vi "Check Lower Warning.vi"(8 "error in (no error)":errorcluster, 10 "Input Values":sgl[](array[numeric]), 11 "AILimitConfig":T1(array[cluster])) -> (0 "error out":errorcluster, 3 "LW Channel":string[](array[string]))   [LabVIEW 2018]
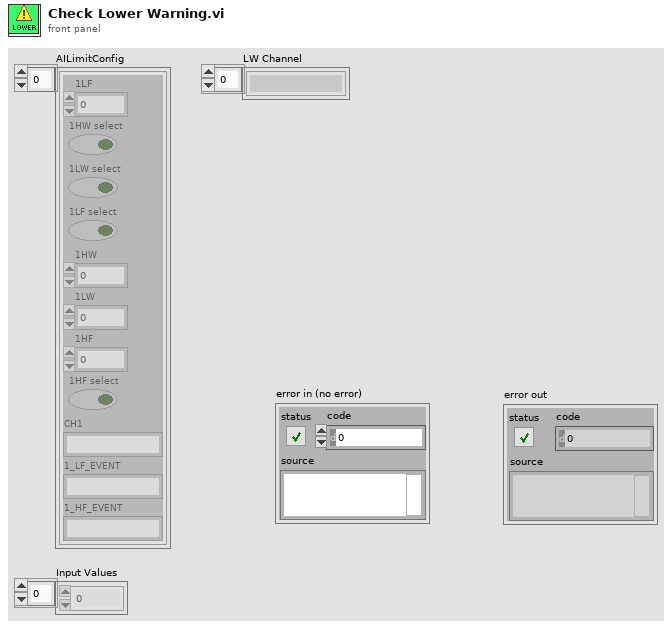
[diagram p1: front panel]
types:
  T1 = cluster{"1LF":dbl, "1HW select":bool, "1LW select":bool, "1LF select":bool, "1HW":dbl, "1LW":dbl, "1HF":dbl, "1HF select":bool, "CH1":string, "1_LF_EVENT":string, "1_HF_EVENT":string}[]
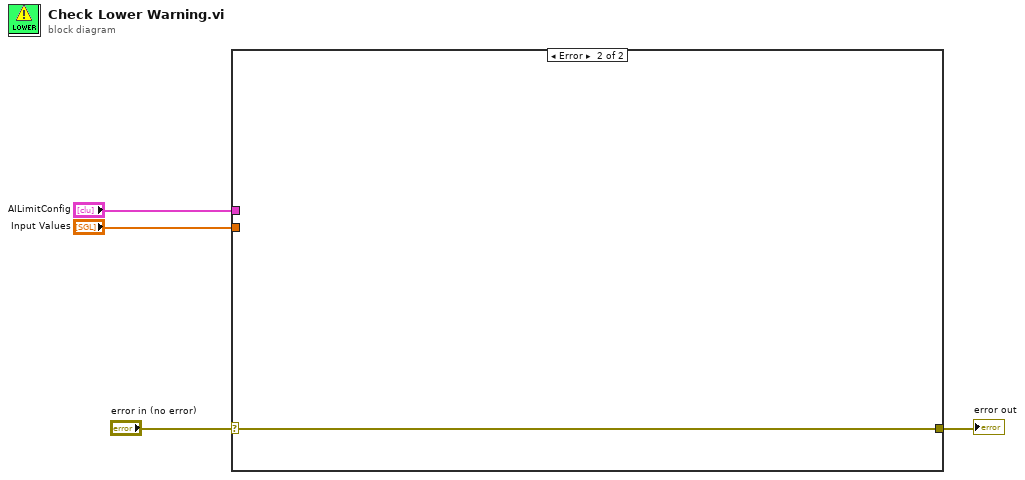
[diagram p0: block diagram]
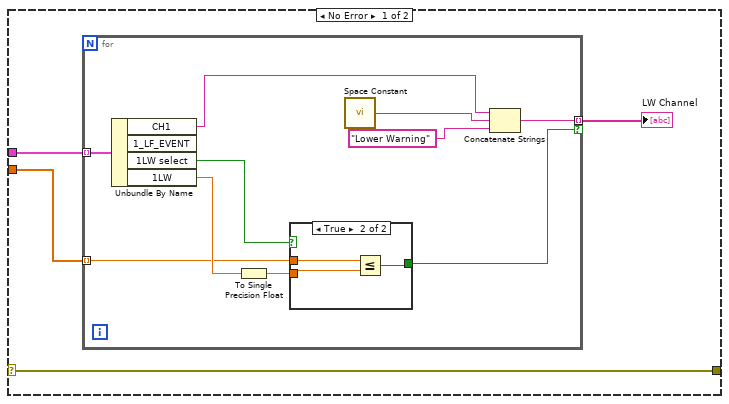
[diagram p2: hidden frame]
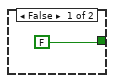
[diagram p3: hidden frame]
diagram:
  n1 = case shown="Error" "error in (no error)" {
    selector: "error in (no error)" -> [w5 w23]
    tunnel: "Input Values" -> [w8 _]
    tunnel: "AILimitConfig" -> [w6 _]
    tunnel: [w5 w23] -> w1
    frame No Error {
      n2 = for {
        tunnel: w6 -> [w18] mode=indexing
        tunnel: w8 -> [w15] mode=indexing
        tunnel: [w11] -> w7 mode=indexing if=w10
        n3 = Unbundle By Name(w18) -> ("CH1"=w12:string, "1LW select"=w17:bool, "1LW"=w16:dbl)  [unwired: 1 out]
        n4 = To Single Precision Float(number=w16) -> (single precision float=w9:sgl)
        n5 = case shown="True" w17 {
          tunnel: w15 -> [_ w22]
          tunnel: w9 -> [_ w21]
          tunnel: [FALSE w20] -> w10
          frame False {
          }
          frame True {
            n6 = Less Or Equal?(x=w22, y=w21) -> (x <= y?=w20:bool)
          }
        }
        n7 = call <vilib>:"Space Constant.vi"() -> ("String"=w14:string)
        n8 = Concatenate Strings(w12, w14, "Lower Warning" ("string")) -> (w11:string)
      }
      "LW Channel" <- w7
    }
    frame Error {
    }
  }
  "error out" <- w1
